vi "Get Object Name.vi"(8 "error in (no error)":errorcluster, 11 "Object":variant) -> (0 "error out":errorcluster, 2 "name":string, 3 "Variant":variant)   [LabVIEW 2019, in "JSON-Schema.lvlib"]
uses:
  JSON-Schema.lvlib
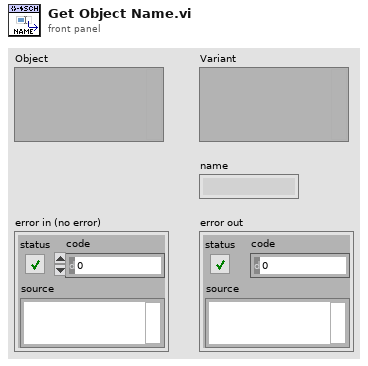
[diagram p1: front panel]
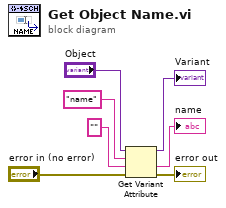
[diagram p0: block diagram]
diagram:
  n1 = Get Variant Attribute(Variant="Object", name="name", default value (empty Variant)="" ("name"), error in="error in (no error)") -> (duplicate Variant=→"Variant":variant, value=→"name":string, error out=→"error out":errorcluster)  [unwired: 1 out]
